vi "REV2mDistanceSensor Get Range.vi"(8 "error in":errorcluster, 9 "Units (Inches)":T4=enum."Inches", 10 "Port":T3=enum."MXP", 11 "REV2mDistanceSensorsArray":T1) -> (0 "error out":errorcluster, 1 "Range":dbl, 2 "Is Valid?":bool, 3 "REV2mDistanceSensorsArray Out":T1)   [LabVIEW 2019, in "DistanceSensorDriver.lvlib"]
uses:
  DistanceSensorDriver.lvlib
  Typedef/Ports.ctl
  Typedef/Units.ctl
  Typedef/Rev2mDistanceSensorsArray.ctl
  Typedef/REV2mDistanceSensorDevRef.ctl
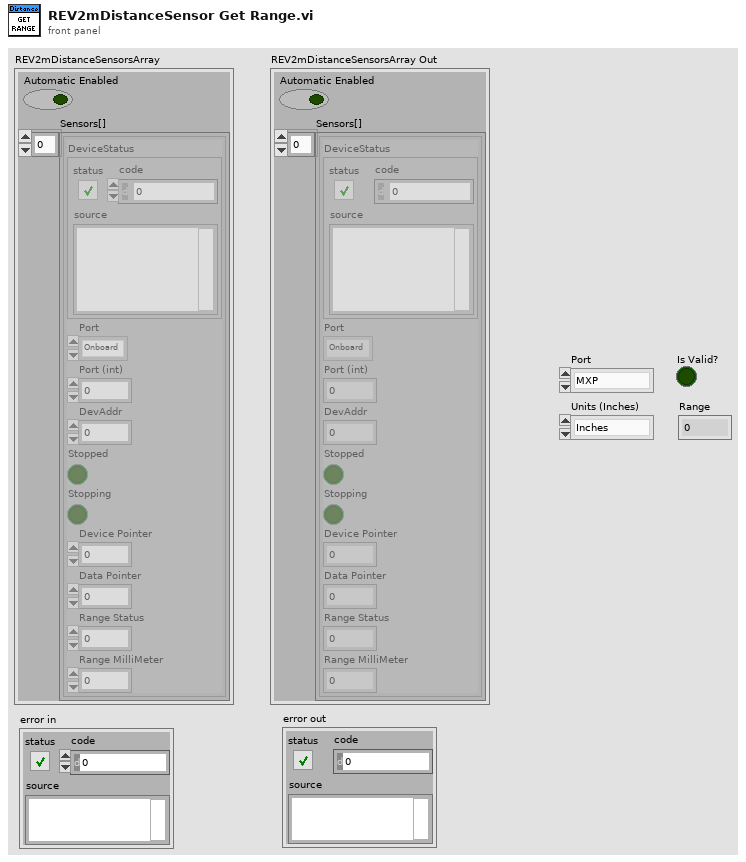
[diagram p1: front panel]
types:
  T1 = typedef "DistanceSensorDriver.lvlib/Rev2mDistanceSensorsArray.ctl" = cluster{"Automatic Enabled":bool, "Sensors[]":T2[]}
  T2 = typedef "DistanceSensorDriver.lvlib/REV2mDistanceSensorDevRef.ctl" = cluster{"DeviceStatus":errorcluster, "Port":T3, "Port (int)":i32, "DevAddr":i32, "Stopped":bool, "Stopping":bool, "Device Pointer":u64, "Data Pointer":u64, "Range Status":u8, "Range MilliMeter":u16}
  T3 = typedef "DistanceSensorDriver.lvlib/Ports.ctl" = enum32{"Onboard", "MXP"}
  T4 = typedef "DistanceSensorDriver.lvlib/Units.ctl" = enum16{"Millimeters", "Inches"}
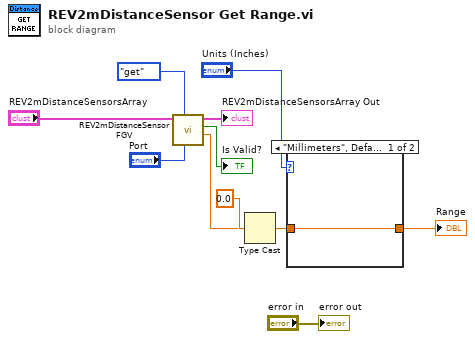
[diagram p0: block diagram]
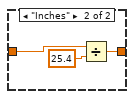
[diagram p2: hidden frame]
diagram:
  n1 = call "REV2mDistanceSensor FGV.vi"("Port"="Port", "Operation"=enum16{"set", "get"}."get", "REV2mDistanceSensorsArray"="REV2mDistanceSensorsArray") -> ("Range"=w2:dbl, "Range Valid"=→"Is Valid?":bool, "REV2mDistanceSensorsArray Out"=→"REV2mDistanceSensorsArray Out":T1)  [unwired: 5 in, 1 out]
  n2 = Type Cast(type=0.0, x=w2) -> (*(type *) &x=w7:dbl)
  n3 = case shown="\"Millimeters\", Default" "Units (Inches)" {
    tunnel: w7 -> [w12 w15]
    tunnel: [w12 w14] -> w10
    frame "Millimeters", Default {
    }
    frame "Inches" {
      n4 = Divide(x=w15, y=25.4) -> (x/y=w14:dbl)
    }
  }
  "Range" <- w10
  "error out" <- "error in"
